vi "未命名 2.vi"(3 "Annulus":T1 {"End Angle" min=-90.0 max=90.0 step=1.0 format="%.2f"; "Start Angle" min=-90.0 max=90.0 step=1.0 format="%.2f"; "Center X" scale=0.0..1024.0}, 10 "铜片有无圆心参数":cluster{"圆环ROI设定":T1, "黑像素个数判定阀值":dbl}={"圆环ROI设定"={"Center X"=1717, "Center Y"=1486, "Inner Radius"=327, "Outer Radius"=1645, "Start Angle"=0.0, "End Angle"=0.0}, "黑像素个数判定阀值"=0.0} {"圆环ROI设定"."End Angle" min=-90.0 max=90.0 step=1.0 format="%.2f"; "圆环ROI设定"."Start Angle" min=-90.0 max=90.0 step=1.0 format="%.2f"; "圆环ROI设定"."Center X" scale=0.0..1024.0}) -> (2 "输出簇 2":cluster{"圆环ROI设定":T1, "黑像素个数判定阀值":dbl} {"圆环ROI设定"."End Angle" min=-90.0 max=90.0 step=1.0 format="%.2f"; "圆环ROI设定"."Start Angle" min=-90.0 max=90.0 step=1.0 format="%.2f"; "圆环ROI设定"."Center X" scale=0.0..1024.0})   [LabVIEW 2017]
panel:
  out "输出簇":T1 {"End Angle" min=-90.0 max=90.0 step=1.0 format="%.2f"; "Start Angle" min=-90.0 max=90.0 step=1.0 format="%.2f"; "Center X" scale=0.0..1024.0}
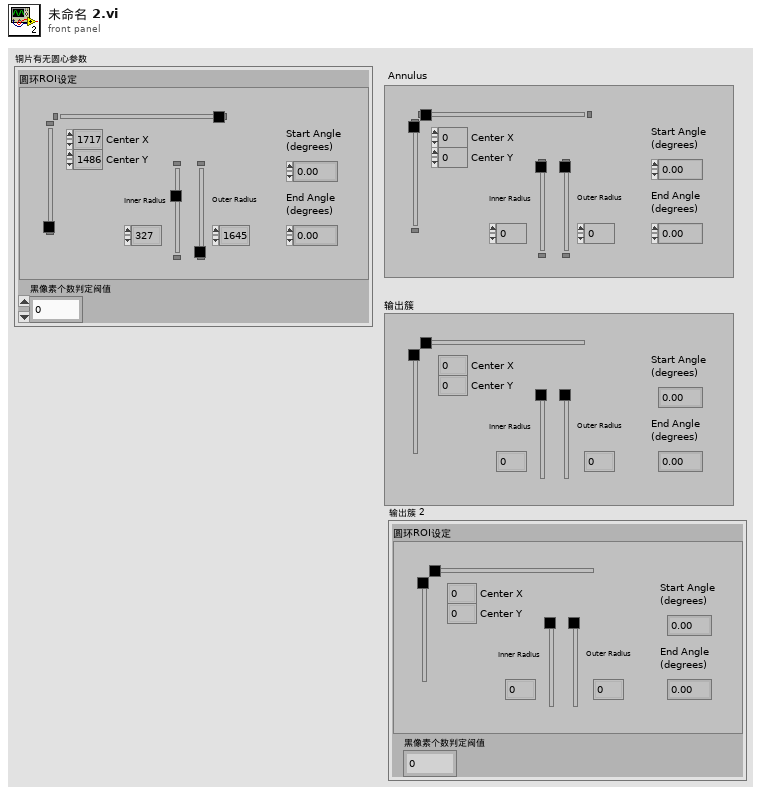
[diagram p1: front panel]
types:
  T1 = typedef "IMAQ Circle" = cluster{"Center X":i32, "Center Y":i32, "Inner Radius":i32, "Outer Radius":i32, "Start Angle":dbl, "End Angle":dbl}
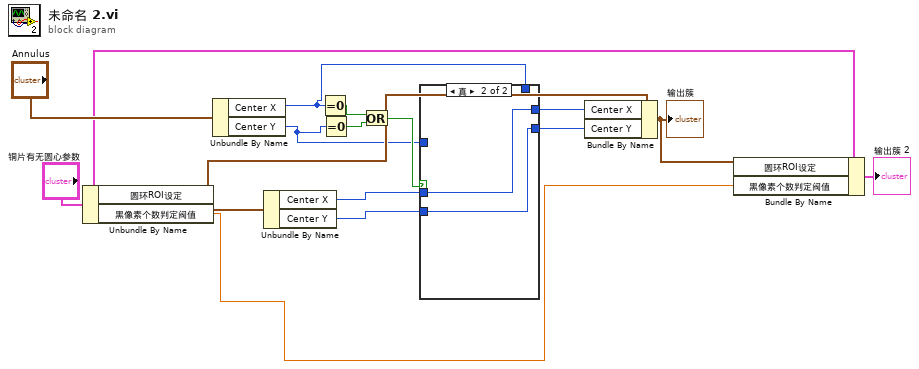
[diagram p0: block diagram]
diagram:
  n1 = Unbundle By Name("铜片有无圆心参数") -> ("圆环ROI设定"=w14:T1, "黑像素个数判定阀值"=w2:dbl)
  n2 = Unbundle By Name("Annulus") -> ("Center X"=w6:i32, "Center Y"=w5:i32)
  n3 = Unbundle By Name(w14) -> ("Center X"=w9:i32, "Center Y"=w7:i32)
  n4 = Equal To 0?(x=w6) -> (x = 0?=w13:bool)
  n5 = Equal To 0?(x=w5) -> (x = 0?=w12:bool)
  n6 = Or(x=w13, y=w12) -> (x .or. y?=w11:bool)
  n7 = case shown="真" w11 {
    tunnel: [w17 w19] -> w10
    tunnel: w9 -> [_ w19]
    tunnel: [w16 w18] -> w8
    tunnel: w7 -> [_ w18]
    tunnel: w6 -> [w17 _]
    tunnel: w5 -> [w16 _]
    frame False {
    }
    frame True {
    }
  }
  n8 = Bundle By Name(cluster=w14, "Center X"=w10, "Center Y"=w8) -> (w3:T1)
  "输出簇" <- w3
  n9 = Bundle By Name(cluster="铜片有无圆心参数", "圆环ROI设定"=w3, "黑像素个数判定阀值"=w2) -> (→"输出簇 2":cluster{"圆环ROI设定":T1, "黑像素个数判定阀值":dbl})
